vi "Set Connected.vi"(8 "error in (no error)":errorcluster, 10 "Connected":bool, 11 "Instrument Properties in":refnum<class "Instrument Properties.lvclass">) -> (0 "error out":errorcluster, 3 "Instrument Properties out":refnum<class "Instrument Properties.lvclass">)   [LabVIEW 2015, in "Instrument.lvlib" / "Instrument Properties.lvclass"]
uses:
  Instrument Properties.lvclass
  Instrument Properties.lvclass/Instrument Properties.ctl
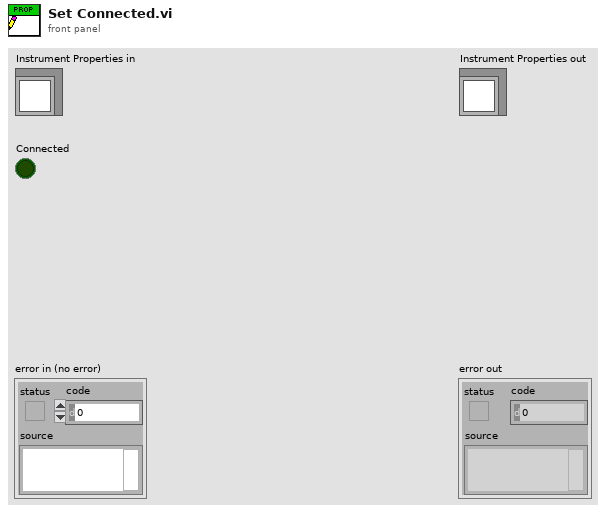
[diagram p1: front panel]
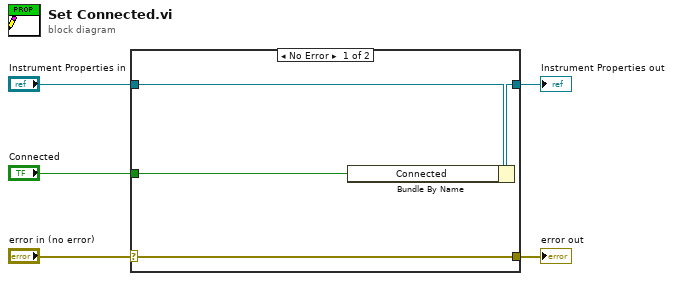
[diagram p0: block diagram]
diagram:
  n1 = case shown="No Error" "error in (no error)" {
    selector: "error in (no error)" -> [w9 w10]
    tunnel: [w9 w10] -> w4
    tunnel: [w7 w11] -> w2
    tunnel: "Instrument Properties in" -> [w8 w11]
    tunnel: "Connected" -> [w6 _]
    frame No Error {
      n2 = Bundle By Name(cluster=w8, "Connected"=w6) -> (w7:refnum<class "Instrument Properties.lvclass">)
    }
    frame Error {
    }
  }
  "error out" <- w4
  "Instrument Properties out" <- w2
